vi "delete Norm.vi"(8 "error in (no error)":errorcluster caption="Fehler (Eingang, kein Fehler)", 10 "id":i32, 11 "Report (Eingang)":refnum<class "Report.lvclass">) -> (0 "error out":errorcluster caption="Fehler (Ausgang)", 3 "Report (Ausgang)":refnum<class "Report.lvclass">)   [LabVIEW 2013, in "DatenKlassen.lvlib" / "Report.lvclass"]
uses:
  Report.lvclass
  Report.lvclass/Report.ctl
  Norm/Norm.lvclass
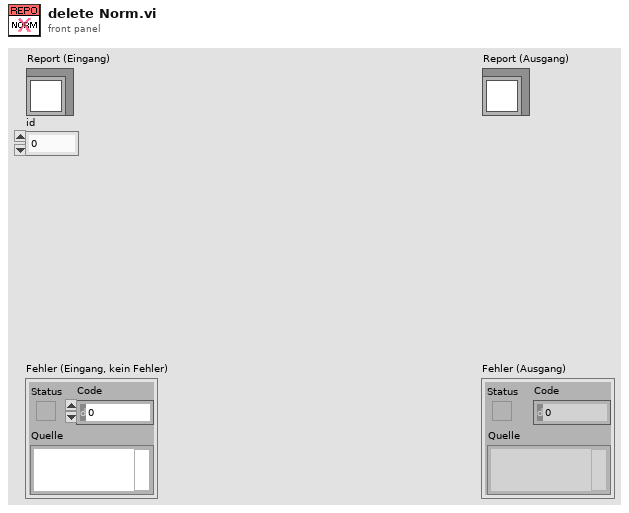
[diagram p1: front panel]
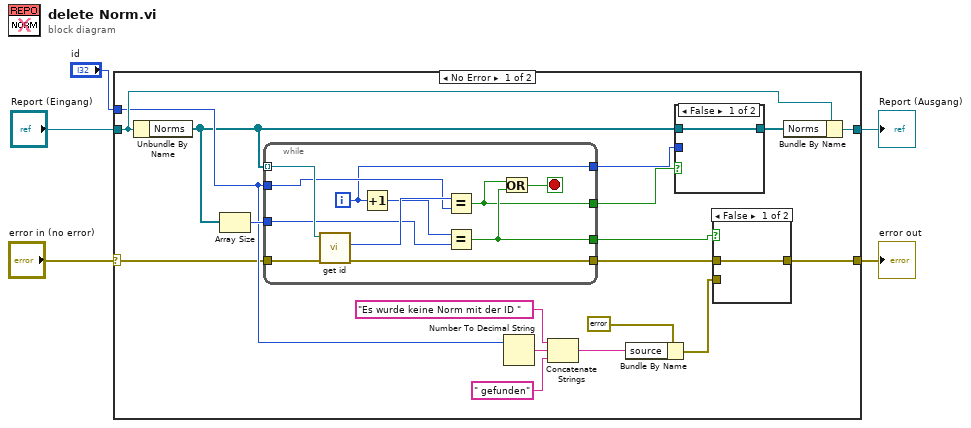
[diagram p0: block diagram]
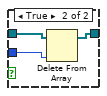
[diagram p2: hidden frame]
diagram:
  n1 = case shown="No Error" "error in (no error)" {
    selector: "error in (no error)" -> [w7 w41]
    tunnel: [w12 w41] -> w4
    tunnel: [w23 w42] -> w2
    tunnel: "Report (Eingang)" -> [w22 w42]
    tunnel: "id" -> [w20 _]
    frame No Error {
      n2 = Unbundle By Name(w22) -> ("Norms"=w9:refnum<class "Norm.lvclass">[])
      n3 = Array Size(array=w9) -> (size(s)=w21:i32)
      n4 = while {
        tunnel: w9 -> [w40] mode=indexing
        tunnel: w20 -> [w38]
        tunnel: w21 -> [w36]
        tunnel: [w34] -> w14
        tunnel: [w33] -> w11
        tunnel: [w32] -> w10
        tunnel: w7 -> [w31]
        tunnel: [w30] -> w6
        i -> [w32]
        stop <- w35 stop-if-true
        n5 = call-dynamic "get id.vi"("error in (no error)"=w31, "Norm (Eingang)"=w40) -> ("error out"=w30:errorcluster, "id"=w39:i32)  [unwired: 7 in, 1 out]
        n6 = Increment(x=w32) -> (x+1=w37:i32)
        n7 = Equal?(x=w39, y=w38) -> (x = y?=w33:bool)
        n8 = Equal?(x=w37, y=w36) -> (x = y?=w34:bool)
        n9 = Or(x=w33, y=w34) -> (x .or. y?=w35:bool)
      }
      n10 = Number To Decimal String(number=w20) -> (decimal integer string=w18:string)  [unwired: 1 in]
      n11 = Concatenate Strings("Es wurde keine Norm mit der ID " ("source"), w18, " gefunden" ("string")) -> (w15:string)
      n12 = Bundle By Name(cluster=errorcluster {"status"=TRUE, "code"=99999, "source"="Es wurde keine Norm mit der ID "} ("error constant"), "source"=w15) -> (w13:errorcluster)
      n13 = case shown="False" w11 {
        tunnel: w10 -> [_ w26]
        tunnel: w9 -> [w24 w27]
        tunnel: [w24 w25] -> w8
        frame False {
        }
        frame True {
          n14 = Delete From Array(array=w27, index=w26) -> (array with subset deleted=w25:refnum<class "Norm.lvclass">[])  [unwired: 1 in, 1 out]
        }
      }
      n15 = case shown="False" w14 {
        tunnel: [w28 w29] -> w12
        tunnel: w13 -> [_ w29]
        tunnel: w6 -> [w28 _]
        frame False {
        }
        frame True {
        }
      }
      n16 = Bundle By Name(cluster=w22, "Norms"=w8) -> (w23:refnum<class "Report.lvclass">)
    }
    frame Error {
    }
  }
  "error out" <- w4
  "Report (Ausgang)" <- w2
